vi "AutonSwitchFile.vi"(9 "Number of Auton Files":dbl, 10 "Auton File":dbl, 11 "Auton Files":string[](array[string])) -> (2 "Current File":string, 3 "Auton Array":dbl[][](array[numeric]))   [LabVIEW 2011]
uses:
  <vilib>/Rock Robotics/WPI/DriverStation/DriverStationLCD/WPI_DriverStationLCDLCDLine.ctl
  <vilib>/Utility/file.llb/Read From Spreadsheet File (DBL).vi
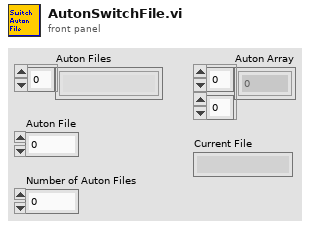
[diagram p1: front panel]
types:
  T1 = typedef "WPI_DriverStationLCDLCDLine.ctl" = enum16{"Main - Line 1", "User - Line 2", "User - Line 3", "User - Line 4", "User - Line 5", "User - Line 6"}
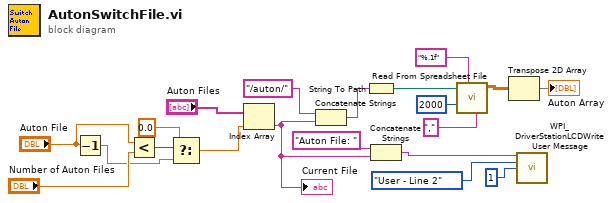
[diagram p0: block diagram]
diagram:
  n1 = Decrement(x="Auton File") -> (x-1=w7:dbl)
  n2 = Less?(x="Auton File", y="Number of Auton Files") -> (x < y?=w3:bool)
  n3 = Select(t=0.0, s=w3, f=w7) -> (s? t:f=w5:dbl)
  n4 = Index Array(array="Auton Files", index=w5) -> (element=w19:string)
  "Current File" <- w19
  n5 = Concatenate Strings("/auton/" ("string"), w19) -> (w11:string)
  n6 = String To Path(string=w11) -> (path=w12:path)
  n7 = Concatenate Strings("Auton File: " ("string"), w19) -> (w20:string)
  n8 = call-poly <vilib>:"Read From Spreadsheet File.vi"("delimiter (\\t)"="," ("delimiter (\\t)"), "format (%.3f)"="%.1f", "number of rows (all:-1)"=2000, "file path (dialog if empty)"=w12) -> ("all rows"=w14:dbl[][])  [unwired: 1 in, 6 out]
  n9 = Transpose 2D Array(2D array=w14) -> (transposed array=→"Auton Array":dbl[][])
  n10 = call <vilib>:"WPI_DriverStationLCDWrite User Message.vi"("line text"=w20, "line"=WPI_DriverStationLCDLCDLine."User - Line 2", "starting column"=i8 1) -> ()  [unwired: 2 in, 11 out]
